vi "Save Data.vi"(8 "error in (no error)":errorcluster, 10 "Numeric":dbl, 11 "CSVV in":refnum<class "CSVV.lvclass">) -> (0 "error out":errorcluster, 3 "Logging out":refnum<class "Logging.lvclass">)   [LabVIEW 2019, in "CSVV.lvlib" / "CSVV.lvclass"]
uses:
  CSVV.lvclass
  E:/7to semestre/instrumentacion virtual/parcial 2/AFTarea/Logging/Logging/Logging.lvclass
  Logging/Logging/Logging.lvclass
  Logging/Logging/Logging.lvclass/Logging.ctl
  <vilib>/Utility/file.llb/Write Delimited Spreadsheet (DBL).vi
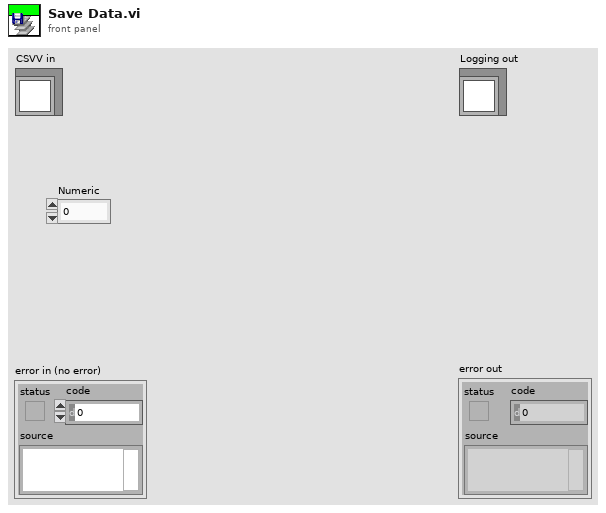
[diagram p1: front panel]
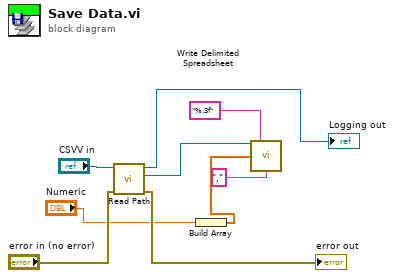
[diagram p0: block diagram]
diagram:
  n1 = call "Read Path.vi"("error in (no error)"="error in (no error)", "Logging in"="CSVV in") -> ("error out"=→"error out":errorcluster, "Path"=w5:path, "Logging out"=→"Logging out":refnum<class "CSVV.lvclass">)  [unwired: 7 in]
  n2 = Build Array("Numeric") -> (w3:dbl[])
  n3 = call-poly <vilib>:"Write Delimited Spreadsheet.vi"("file path (dialog if empty)"=w5, "format (%.3f)"="%.3f", "1D data"=w3, "delimiter (\\t)"="," ("delimiter (\\t)")) -> ()  [unwired: 10 in, 2 out]
